vi "_Send Command.vi"(8 "error in (no error)":errorcluster, 9 "Query? (F)":bool, 10 "Command":string, 11 "VISA resource name":refnum<visa-resource-name>="GPIB0::23::INSTR") -> (0 "error out":errorcluster, 2 "Response":string, 3 "VISA resource name out":refnum<visa-resource-name>)   [LabVIEW 2012, in "SR400.lvlib"]
uses:
  SR400.lvlib
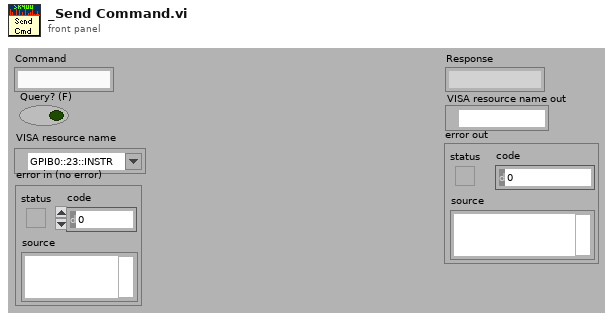
[diagram p1: front panel]
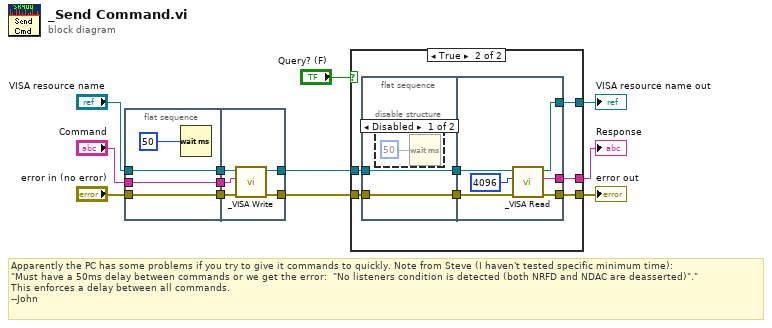
[diagram p0: block diagram]
diagram:
  # "Apparently the PC has some problems if you try to give it commands to quickly. Note from Steve (I haven't tested specific minimum time): \n\"Must have a 50ms delay between commands or we get the error:  \"No listeners condition is detected (both NRFD and NDAC are deasserted)\".\"\nThis enforces a delay between all commands. \n--John"
  n1 = flat-sequence {
    tunnel: "error in (no error)" -> [w14]
    tunnel: "VISA resource name" -> [w15]
    tunnel: "Command" -> [w16]
    tunnel: [w16] -> w9
    tunnel: [w15] -> w8
    tunnel: [w14] -> w7
    tunnel: w9 -> [w19]
    tunnel: w8 -> [w20]
    tunnel: w7 -> [w21]
    tunnel: [w18] -> w5
    tunnel: [w17] -> w4
    frame #0 {
      n2 = Wait (ms)(milliseconds to wait=50) -> ()  [unwired: 1 out]
    }
    frame #1 {
      n3 = call "_VISA Write.vi"("error in (no error)"=w21, "write buffer"=w19, "VISA resource name"=w20) -> ("error out"=w17:errorcluster, "VISA resource name out"=w18:refnum<visa-resource-name>)  [unwired: 7 out]
    }
  }
  n4 = case shown="True" "Query? (F)" {
    tunnel: [_ w30] -> w2
    tunnel: w4 -> [w23 w29]
    tunnel: w5 -> [w22 w28]
    tunnel: [w23 w27] -> w1
    tunnel: [w22 w26] -> w3
    frame False {
    }
    frame True {
      n5 = flat-sequence {
        tunnel: w28 -> [w31]
        tunnel: w29 -> [w32]
        tunnel: [w32] -> w25
        tunnel: [w31] -> w24
        tunnel: [w39] -> w30
        tunnel: [w35] -> w27
        tunnel: [w34] -> w26
        tunnel: w25 -> [w38]
        tunnel: w24 -> [w37]
        frame #0 {
          n6 = disable-structure shown="Disabled" {
            frame Disabled {
              n7 = Wait (ms)(milliseconds to wait=50) -> ()  [unwired: 1 out]
            }
            frame Enabled {
            }
          }
        }
        frame #1 {
          n8 = call "_VISA Read.vi"("error in (no error)"=w38, "byte count"=u32 4096, "VISA resource name"=w37) -> ("error out"=w35:errorcluster, "read buffer"=w39:string, "VISA resource name out"=w34:refnum<visa-resource-name>)  [unwired: 6 out]
        }
      }
    }
  }
  "Response" <- w2
  "VISA resource name out" <- w3
  "error out" <- w1
